vi "waitForModbusIRQs.vi"(8 "error in (no error)":errorcluster, 10 "Timeout (ms)":i32, 11 "Model in":refnum<class "Model.lvclass">) -> (0 "error out":errorcluster, 3 "Model out":refnum<class "Model.lvclass">)   [LabVIEW 2016, in "Model.lvclass"]
uses:
  Model.lvclass
  Model.lvclass/Model.ctl
  Resources/FPGA/FPGA.lvclass
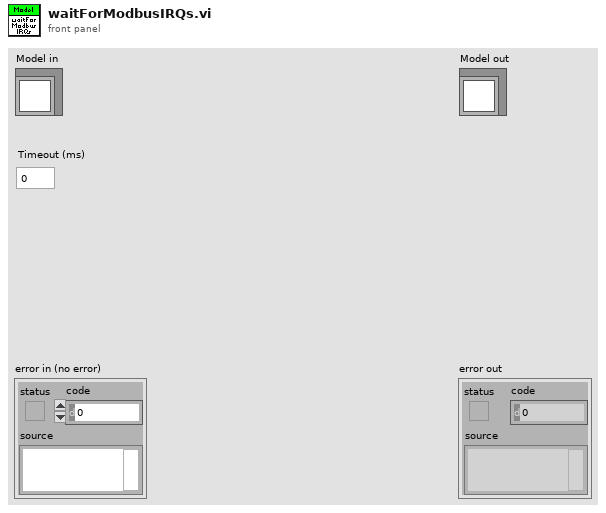
[diagram p1: front panel]
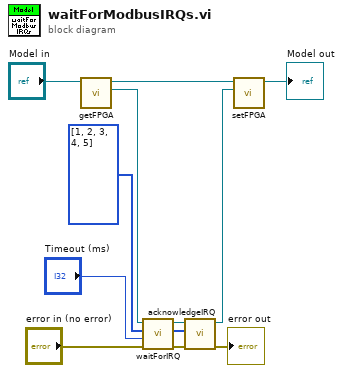
[diagram p0: block diagram]
diagram:
  n1 = call "getFPGA.vi"("Model in"="Model in") -> ("FPGA"=w10:refnum<class "FPGA.lvclass">, "Model out"=w11:refnum<class "Model.lvclass">)  [unwired: 9 in]
  n2 = call "waitForIRQ.vi"("error in (no error)"="error in (no error)", "Timeout (ms)"="Timeout (ms)", "IRQs in"=i32[] [1, 2, 3, 4, 5], "FPGA in"=w10) -> ("error out"=w5:errorcluster, "IRQs out"=w4:i32[], "FPGA out"=w9:refnum<class "FPGA.lvclass">)  [unwired: 4 in, 1 out]
  n3 = call "acknowledgeIRQ.vi"("error in (no error)"=w5, "IRQs"=w4, "FPGA in"=w9) -> ("error out"=→"error out":errorcluster, "FPGA out"=w8:refnum<class "FPGA.lvclass">)  [unwired: 7 in]
  n4 = call "setFPGA.vi"("FPGA"=w8, "Model in"=w11) -> ("Model out"=→"Model out":refnum<class "Model.lvclass">)  [unwired: 9 in]
